vi "Auton Script Builder.vi"(10 "Export?":bool) -> (2 "Export Successful":bool)   [LabVIEW 2017]
uses:
  Robot Global Data.vi
  <vilib>/Utility/file.llb/Read Delimited Spreadsheet (DBL).vi
  <vilib>/Utility/file.llb/Write Delimited Spreadsheet (DBL).vi
panel:
  out "error out 2":errorcluster
  out "error out":errorcluster
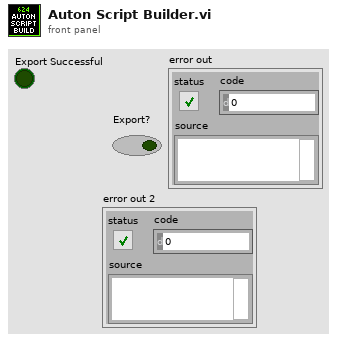
[diagram p1: front panel]
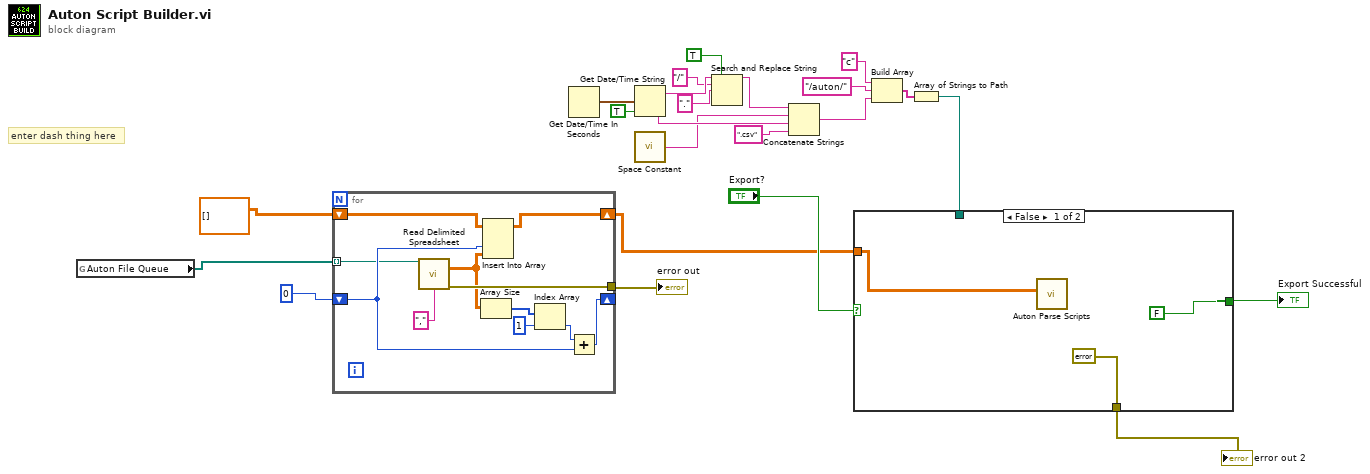
[diagram p0: block diagram]
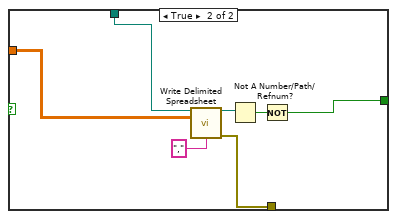
[diagram p2: hidden frame]
diagram:
  # "enter dash thing here"
  n1 = global read "Robot Global Data.vi" "Auton File Queue"() -> (w3:path[])
  n2 = for {
    shift-right: [w33] -> w4
    shift-left: dbl[][] [] -> [w34]
    tunnel: [w31] -> w5
    shift-right: [w26] -> _
    shift-left: 0 -> [w25]
    tunnel: w3 -> [w24] mode=indexing
    n3 = call-poly <vilib>:"Read Delimited Spreadsheet.vi"("file path (dialog if empty)"=w24, "delimiter (\\t)"="," ("delimiter (\\t)")) -> ("all rows"=w30:dbl[][], "error out"=w31:errorcluster)  [unwired: 8 in, 4 out]
    n4 = Array Size(array=w30) -> (size(s)=w29:i32[])
    n5 = Insert Into Array(array=w34, index (col)=w25, new element=w30) -> (w33:dbl[][])  [unwired: 1 in]
    n6 = Index Array(array=w29, index=1) -> (element=w27:i32)
    n7 = Add(x=w27, y=w25) -> (x+y=w26:i32)
  }
  "error out" <- w5
  n8 = Get Date/Time In Seconds() -> (seconds since 1Jan1904=w20:timestamp)
  n9 = Get Date/Time String(seconds (now)=w20, want seconds? (F)=TRUE) -> (date string=w15:string, time string=w18:string)  [unwired: 1 in]
  n10 = call <vilib>:"Space Constant.vi"() -> ("String"=w10:string)
  n11 = Search and Replace String(replace all?=TRUE ("replace all? (F)"), input string=w15, search string="/", replace string="." ("replace string (\"\")")) -> (result string=w11:string)  [unwired: 4 in, 3 out]
  n12 = Concatenate Strings(w11, w10, w18, ".csv" ("element")) -> (w16:string)
  n13 = Build Array("c", "/auton/", w16) -> (w21:string[])
  n14 = Array of Strings to Path(0:w21) -> (2:w9:path)  [unwired: 1 in]
  n15 = case shown="False" "Export?" {
    tunnel: w9 -> [_ w41]
    tunnel: w4 -> [w35 w40]
    tunnel: [errorcluster {"status"=FALSE, "code"=0, "source"=""} ("error out") w38] -> w2
    tunnel: [FALSE w39] -> w1
    frame False {
      n16 = call "Auton Parse Scripts.vi"("Array"=w35) -> ()  [unwired: 11 in]
    }
    frame True {
      n17 = call-poly <vilib>:"Write Delimited Spreadsheet.vi"("file path (dialog if empty)"=w41, "2D data"=w40, "delimiter (\\t)"="," ("delimiter (\\t)")) -> ("new file path (Not A Path if cancelled)"=w43:path, "error out"=w38:errorcluster)  [unwired: 11 in]
      n18 = Not A Number/Path/Refnum?(number/path/refnum=w43) -> (NaN/Path/Refnum?=w42:bool)
      n19 = Not(x=w42) -> (.not. x?=w39:bool)
    }
  }
  "error out 2" <- w2
  "Export Successful" <- w1
